vi "Initialize.vi"(8 "error in (no error)":errorcluster, 11 "Cypress CY8CKIT-059 in":refnum<class "Cypress CY8CKIT-059.lvclass">) -> (0 "error out":errorcluster, 2 "Connected?":bool, 3 "Cypress CY8CKIT-059 out":refnum<class "Cypress CY8CKIT-059.lvclass">)   [LabVIEW 2020, in "Cypress CY8CKIT-059.lvclass"]
doc: "Initialize a device."
uses:
  Cypress CY8CKIT-059.lvclass
  Cypress CY8CKIT-059.lvclass/Cypress CY8CKIT-059.ctl
  79f80230-c24a-40c7-9611-75f6acc1e763.vi
  Read Serial Port.vi
  Write Serial Port.vi
  <vilib>/Instr/_visa.llb/VISA Configure Serial Port (Instr).vi
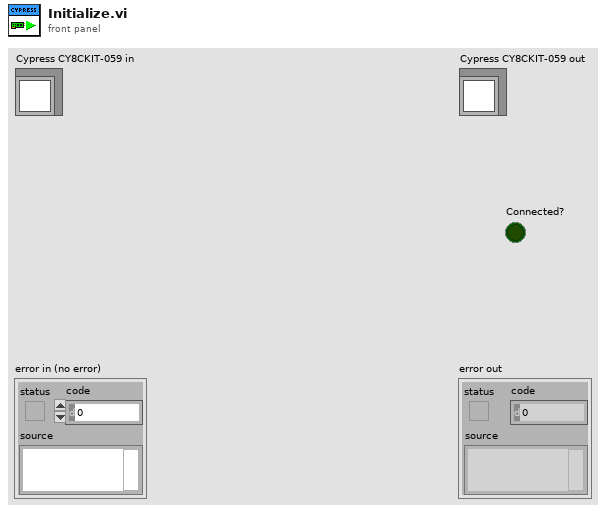
[diagram p1: front panel]
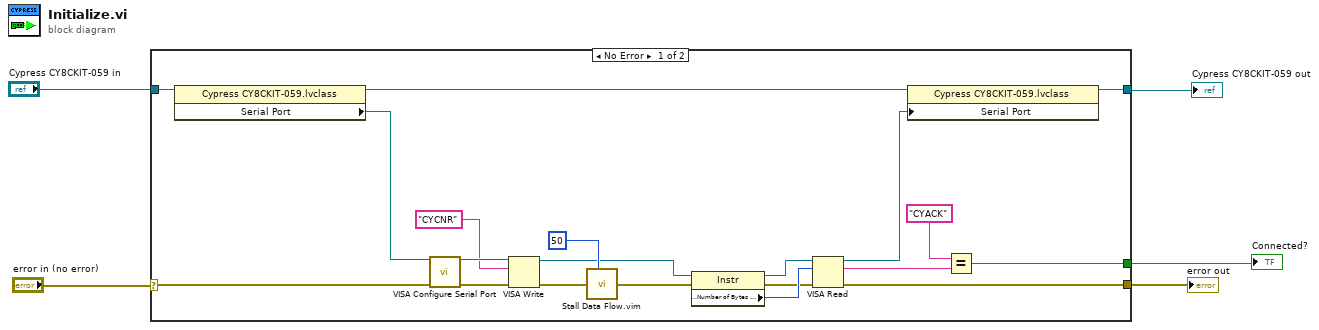
[diagram p0: block diagram]
diagram:
  n1 = case shown="No Error" "error in (no error)" {
    selector: "error in (no error)" -> [w23 w26]
    tunnel: [w21 w27] -> w4
    tunnel: "Cypress CY8CKIT-059 in" -> [w25 w27]
    tunnel: [w17 w26] -> w2
    tunnel: [w12 _] -> w1
    frame No Error {
      n2 = property class="Cypress CY8CKIT-059.lvclass"(reference=w25) -> (reference out=w24:refnum<class "Cypress CY8CKIT-059.lvclass">, "Serial Port"=w22:refnum<visa-resource-name>)  [unwired: 1 in, 1 out]
      n3 = call-poly "VISA Configure Serial Port"("VISA resource name"=w22, "error in (no error)"=w23) -> ("VISA resource name out"=w19:refnum<visa-resource-name>, "error out"=w20:errorcluster)  [unwired: 12 in]
      n4 = VISA Write(VISA resource name=w19, write buffer="CYCNR", error in (no error)=w20) -> (VISA resource name out=w10:refnum<visa-resource-name>, error out=w16:errorcluster)  [unwired: 1 out]
      n5 = call "Stall Data Flow.vim"("value in"=w16, "milliseconds to wait"=u32 50) -> ("value out"=w6:errorcluster)  [unwired: 1 out]
      n6 = property class="Instr"(reference=w10, error in=w6) -> (reference out=w9:refnum<visa-resource-name>, error out=w7:errorcluster, "Serial Settings:Number of Bytes at Serial Port"=w8:u32)
      n7 = VISA Read(VISA resource name=w9, byte count=w8, error in (no error)=w7) -> (VISA resource name out=w11:refnum<visa-resource-name>, read buffer=w14:string, error out=w17:errorcluster)  [unwired: 1 out]
      n8 = property class="Cypress CY8CKIT-059.lvclass"(reference=w24, "Serial Port"=w11) -> (reference out=w21:refnum<class "Cypress CY8CKIT-059.lvclass">)  [unwired: 1 in, 1 out]
      n9 = Equal?(x="CYACK", y=w14) -> (x = y?=w12:bool)
    }
    frame Error {
    }
  }
  "error out" <- w2
  "Cypress CY8CKIT-059 out" <- w4
  "Connected?" <- w1
